vi "Write DoW.vi"(8 "error in (no error)":errorcluster, 10 "DoW":T1, 11 "Daily in":refnum<class "Daily.lvclass">) -> (0 "error out":errorcluster, 3 "Daily out":refnum<class "Daily.lvclass">)   [LabVIEW 2020, in "Daily.lvclass"]
uses:
  Daily.lvclass
  Daily.lvclass/Daily.ctl
  Daily DoW TYP.ctl
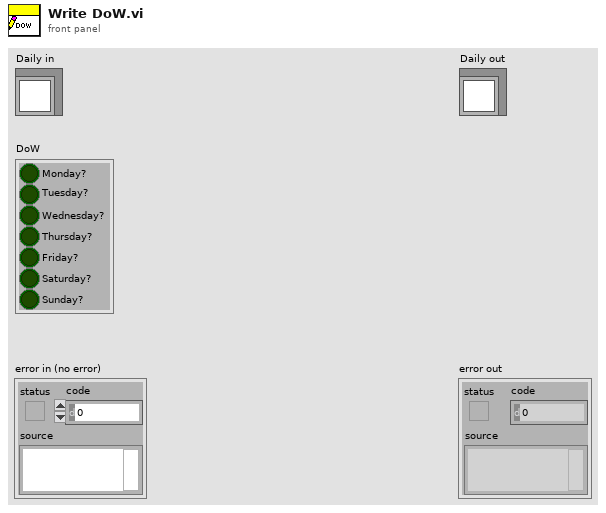
[diagram p1: front panel]
types:
  T1 = typedef "Daily.lvclass/Daily DoW TYP.ctl" = cluster{"Monday?":bool, "Tuesday?":bool, "Wednesday?":bool, "Thursday?":bool, "Friday?":bool, "Saturday?":bool, "Sunday?":bool}
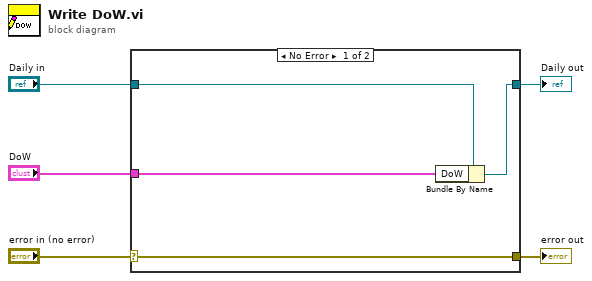
[diagram p0: block diagram]
diagram:
  n1 = case shown="No Error" "error in (no error)" {
    selector: "error in (no error)" -> [w9 w10]
    tunnel: [w9 w10] -> w4
    tunnel: [w7 w11] -> w2
    tunnel: "Daily in" -> [w8 w11]
    tunnel: "DoW" -> [w6 _]
    frame No Error {
      n2 = Bundle By Name(cluster=w8, "DoW"=w6) -> (w7:refnum<class "Daily.lvclass">)
    }
    frame Error {
    }
  }
  "error out" <- w4
  "Daily out" <- w2
